vi "Generate skewed triangular waveform.vi"(4 "Duty cycle (%)":dbl, 5 "Offset":dbl, 6 "sampling info":cluster{"Fs":dbl, "#s":dbl}={"Fs"=1000.0, "#s"=1000.0} {"Fs" format="%.2p"}, 8 "error in (no error)":errorcluster, 9 "Phase":dbl, 10 "Amplitude":dbl, 11 "Frequency":dbl) -> (0 "error out":errorcluster, 3 "Waveform":waveform(dbl))   [LabVIEW 2012]
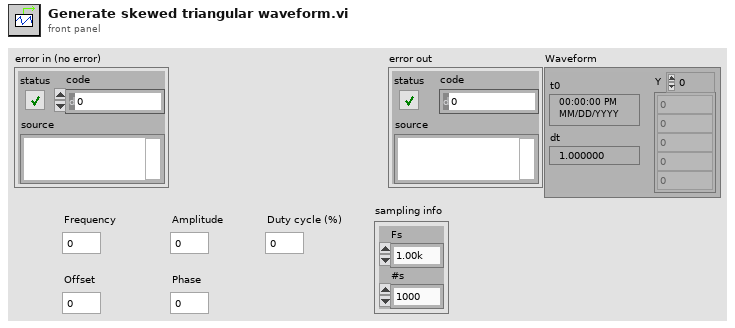
[diagram p1: front panel]
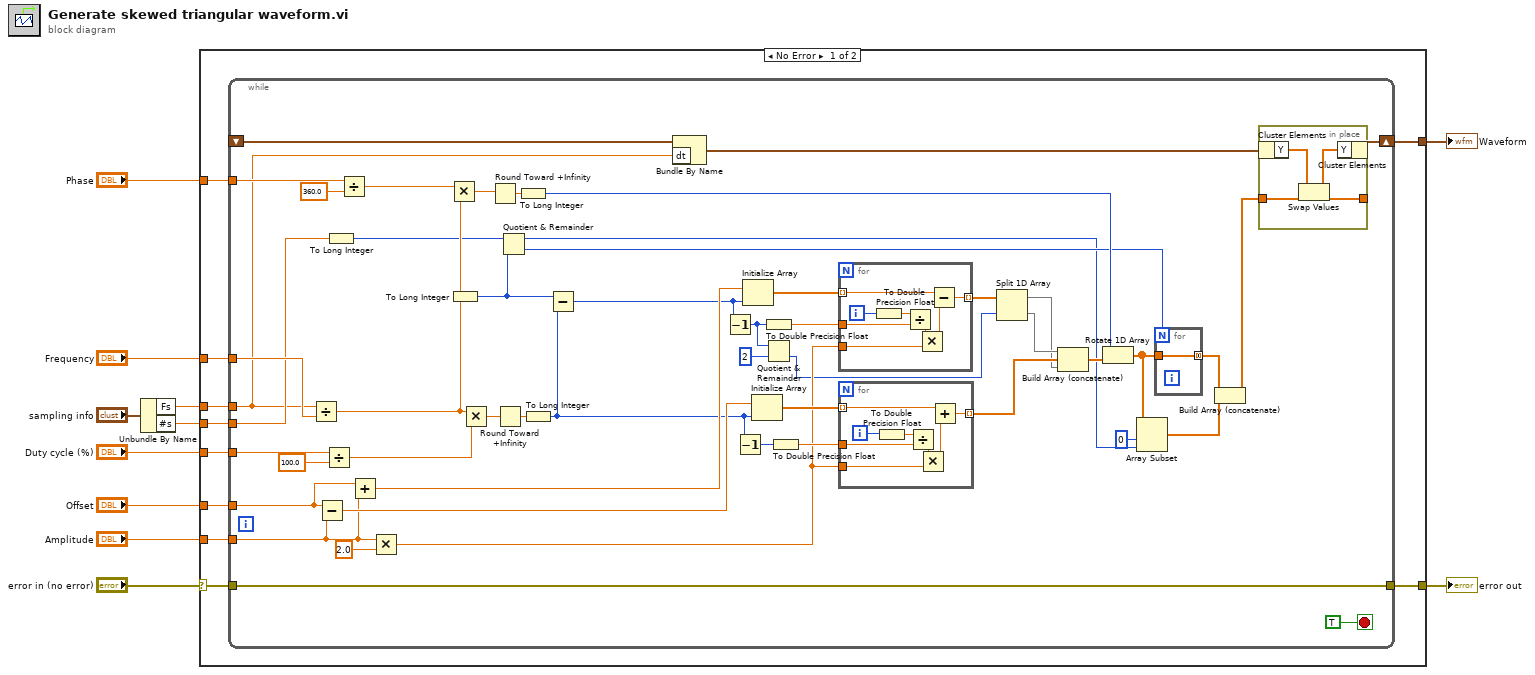
[diagram p0: block diagram]
diagram:
  n1 = Unbundle By Name("sampling info") -> ("Fs"=w4:dbl, "#s"=w7:dbl)
  n2 = case shown="No Error" "error in (no error)" {
    selector: "error in (no error)" -> [w20 w93]
    tunnel: [w12 w93] -> w10
    tunnel: [w21 _] -> w9
    tunnel: w7 -> [w19 _]
    tunnel: "Duty cycle (%)" -> [w18 _]
    tunnel: "Frequency" -> [w17 _]
    tunnel: w4 -> [w16 _]
    tunnel: "Amplitude" -> [w15 _]
    tunnel: "Offset" -> [w14 _]
    tunnel: "Phase" -> [w13 _]
    frame No Error {
      n3 = while {
        shift-right: [w64] -> w21
        shift-left: _ -> [w70]
        tunnel: w20 -> [w28]
        tunnel: w19 -> [w39]
        tunnel: w18 -> [w67]
        tunnel: w17 -> [w63]
        tunnel: w16 -> [w29]
        tunnel: w15 -> [w55]
        tunnel: w14 -> [w58]
        tunnel: w13 -> [w47]
        tunnel: [w28] -> w12
        stop <- TRUE stop-if-true
        n4 = Divide(x=w29, y=w63) -> (x/y=w41:dbl)
        n5 = Subtract(x=w58, y=w55) -> (x-y=w59:dbl)
        n6 = Divide(x=w67, y=100.0) -> (x/y=w68:dbl)
        n7 = To Long Integer(number=w39) -> (32bit integer=w37:i32)
        n8 = Divide(x=w47, y=360.0) -> (x/y=w40:dbl)
        n9 = Add(x=w58, y=w55) -> (x+y=w57:dbl)
        n10 = Multiply(x=w55, y=2.0) -> (x*y=w49:dbl)
        n11 = Multiply(x=w40, y=w41) -> (x*y=w44:dbl)
        n12 = To Long Integer(number=w41) -> (32bit integer=w38:i32)
        n13 = Multiply(x=w41, y=w68) -> (x*y=w62:dbl)
        n14 = Round Toward +Infinity(x=w44) -> (ceil(x): smallest int >= x=w45:dbl)
        n15 = Round Toward +Infinity(x=w62) -> (ceil(x): smallest int >= x=w69:dbl)
        n16 = Quotient & Remainder(x=w37, y=w38) -> (x-y*floor(x/y)=w34:i32, floor(x/y)=w36:i32)
        n17 = To Long Integer(number=w45) -> (32bit integer=w42:i32)
        n18 = To Long Integer(number=w69) -> (32bit integer=w56:i32)
        n19 = Subtract(x=w38, y=w56) -> (x-y=w53:i32)
        n20 = Bundle By Name(cluster=w70, "dt"=w29) -> (w65:waveform(dbl))
        n21 = Decrement(x=w53) -> (x-1=w26:i32)
        n22 = Decrement(x=w56) -> (x-1=w52:i32)
        n23 = Initialize Array(w57, w53) -> (w60:dbl[])
        n24 = Initialize Array(w59, w56) -> (w61:dbl[])
        n25 = To Double Precision Float(number=w26) -> (double precision float=w50:dbl)
        n26 = Quotient & Remainder(x=w26, y=2) -> (floor(x/y)=w24:i32)  [unwired: 1 out]
        n27 = To Double Precision Float(number=w52) -> (double precision float=w51:dbl)
        n28 = for {
          tunnel: w60 -> [w74] mode=indexing
          tunnel: w50 -> [w78]
          tunnel: w49 -> [w77]
          tunnel: [w73] -> w27 mode=indexing
          i -> [w80]
          n29 = To Double Precision Float(number=w80) -> (double precision float=w79:dbl)
          n30 = Divide(x=w79, y=w78) -> (x/y=w76:dbl)
          n31 = Multiply(x=w76, y=w77) -> (x*y=w75:dbl)
          n32 = Subtract(x=w74, y=w75) -> (x-y=w73:dbl)
        }
        n33 = for {
          tunnel: w61 -> [w83] mode=indexing
          tunnel: w51 -> [w86]
          tunnel: w49 -> [w84]
          tunnel: [w81] -> w48 mode=indexing
          i -> [w88]
          n34 = To Double Precision Float(number=w88) -> (double precision float=w87:dbl)
          n35 = Divide(x=w87, y=w86) -> (x/y=w85:dbl)
          n36 = Multiply(x=w85, y=w84) -> (x*y=w82:dbl)
          n37 = Add(x=w83, y=w82) -> (x+y=w81:dbl)
        }
        n38 = Split 1D Array(array=w27, index=w24) -> (first subarray=w22:dbl[], second subarray=w23:dbl[])
        n39 = Build Array (concatenate)(w23, w48, w22) -> (w43:dbl[])
        n40 = Rotate 1D Array(1:w43, 2:w42) -> (0:w35:dbl[])
        n41 = Array Subset(array=w35, index=0, length=w34) -> (w32:dbl[])
        n42 = for {
          N: w36 -> [_]
          tunnel: w35 -> [w72]
          tunnel: [w72] -> w31 mode=concatenating
        }
        n43 = Build Array (concatenate)(w31, w32) -> (w30:dbl[])
        n44 = in-place {
          in-place-border: [w90] -> _
          in-place-border: w30 -> [w89]
          n45 = in-place-cluster #1(w65) -> ("Y"=w92:dbl[])
          n46 = Swap Values(12:w92, 14:w89) -> (1:w91:dbl[], 3:w90:dbl[])  [unwired: 1 in]
          n47 = in-place-cluster #1("Y"=w91) -> (w64:waveform(dbl))
        }
      }
    }
    frame Error {
    }
  }
  "error out" <- w10
  "Waveform" <- w9
